vi "HEWH Test Without Saving.vi"(8 "Error In":errorcluster, 10 "State Input":string="Add Final Data C", 11 "Updated File Path C":T1) -> (0 "Error Out":errorcluster, 3 "SM States":string)   [LabVIEW 2020]
uses:
  Utility/Save File/File Setup (Public)/Type Definition/Save File DOE File Path Control.ctl
  Utility/Save File/File Setup (Public)/Type Definition/Save File DOE Data Save Filepaths.ctl
  Utility/Save File/File Setup.lvlib
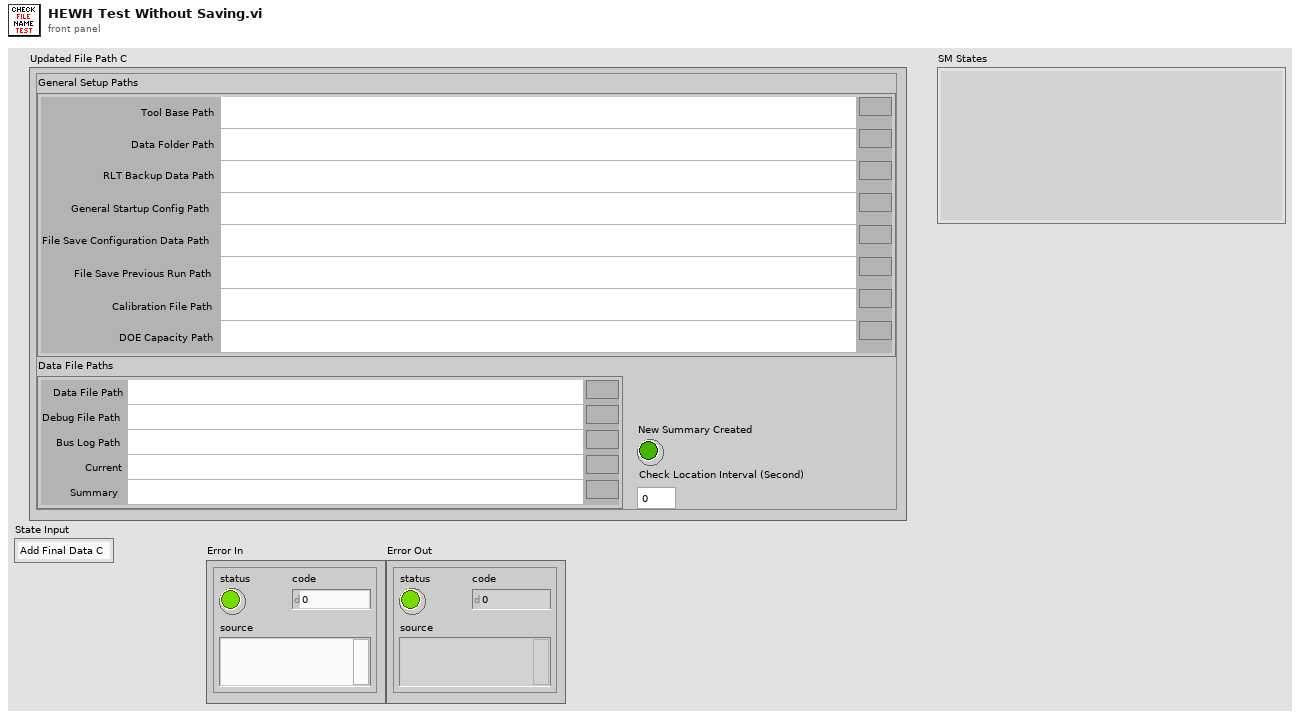
[diagram p1: front panel]
types:
  T1 = typedef "File Setup.lvlib/Save File DOE File Path Control.ctl" = cluster{"General Setup Paths":cluster{"Calibration File Path":path, "DOE Capacity Path":path, "Data Folder Path":path, "RLT Backup Data Path":path, "Tool Base Path":path, "General Startup Config Path":path, "File Save Previous Run Path":path, "File Save Configuration Data Path":path}, "Data File Paths":T2, "New Summary Created":bool, "Check Location Interval (Second)":i32}
  T2 = typedef "File Setup.lvlib/Save File DOE Data Save Filepaths.ctl" = cluster{"Data File Path":path, "Debug File Path":path, "Bus Log Path":path, "Current":path, "Summary":path}
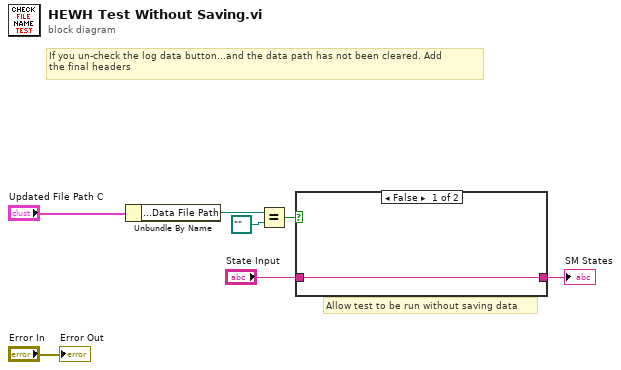
[diagram p0: block diagram]
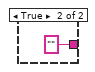
[diagram p2: hidden frame]
diagram:
  # "If you un-check the log data button...and the data path has not been cleared. Add \nthe final headers"
  # "Allow test to be run without saving data"
  n1 = Unbundle By Name("Updated File Path C") -> ("Data File Paths.Data File Path"=w5:path)
  n2 = Equal?(x=w5, y=path "") -> (x = y?=w7:bool)
  n3 = case shown="False" w7 {
    tunnel: [w8 "" ("State(s) in Front (\"\")")] -> w3
    tunnel: "State Input" -> [w8 _]
    frame False {
    }
    frame True {
    }
  }
  "SM States" <- w3
  "Error Out" <- "Error In"
